vi "Global1.vi"() -> ()   [LabVIEW 2026]
doc: "A global variable which contains communication setup information."
uses:
  Available DLLs.ctl
  Available DLL interfaces.ctl
  Available interfaces.ctl
  Termination character.ctl
  Syntax.ctl
panel:
  in  "DLL path":path
  in  "Error Check":bool[](array[boolean])
  in  "PI Semaphore":string[](array[string])
  out "Log file ref. no":refnum<file>
  in  "Logging mode":bool
  in  "Syntax":T1[](array[typedef])
  in  "Termination character":T2[](array[typedef])
  out "VISA Resource name":refnum<visa-resource-name>[](array[refnum])
  in  "TCP/IP Configuration":T3(array[cluster])
  in  "Bit settings and parity":T4(array[cluster]) {"data bits" min=5 max=8 step=1}
  in  "Flow control":T5(array[cluster]) {"parity error byte" format="%.0x"; "XON byte" format="%.0x"; "XOFF byte" format="%.0x"}
  in  "Interface configuration":T7(array[cluster]) {"Interface" items=["RS232", "GPIB", "DLL", "TCP-IP", "USB", "Analog"]; "RS232 Portnumber" items=["COM1", "COM2", "COM3", "COM4", "COM5", "COM6", "COM7", "COM8", "COM9", "COM10", "COM11", "COM12", "COM13", "COM14", "COM15", "COM16", "COM17", "COM18", "COM19", "COM20", "COM21", "COM22", "COM23", "COM24", "COM25", "COM26", "COM27", "COM28", "COM29", "COM30"]}
  in  "DLL Interface\nConfiguration":T10(array[cluster]) {"DLL for Device" items=["C-843", "C-844", "E-710", "C-843.PM", "C-865", "E-761", "Mercury", "E-755", "E-753", "C-866", "E-712", "E-725", "E-861", "C-867", "E-517", "E-816", "E-709", "PI_GCS2_DLL", "HydraPollux"]; "DLL Interface" items=["RS232", "GPIB", "Board", "TCP-IP", "USB", "RS232_DC", "USB_DC", "TCPIP_DC"]}
  in  "DLL device ID's":i32[](array[numeric])
  in  "Number of\nsystems":i32 min=0 max=20 step=1
  # "Global 1 is a global variable which contains communication setup information."
  # "RMO, GKo, 07/12/18"
  # "TCP/IP:"
  # "General:"
  # "RS232:"
  # "GPIB:"
  # "DLL:"
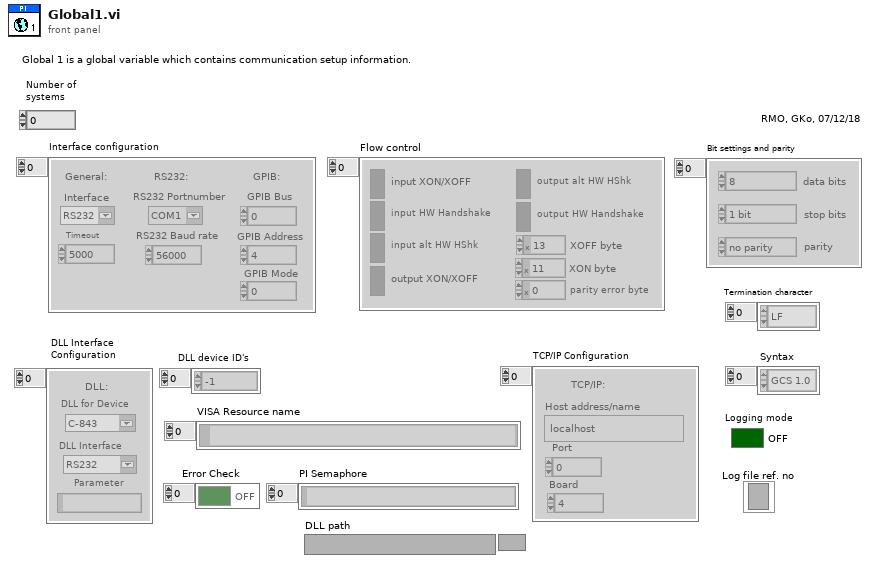
[diagram p1: front panel]
types:
  T1 = typedef "Syntax.ctl" = enum16{"GCS 1.0", "GCS 2.0", "GCS 3.0"}
  T2 = typedef "Termination character.ctl" = enum16{"LF", "CR", "LFCR", "CRLF"}
  T3 = cluster{"Host address/name":string, "Port":i32, "Board":i32}[]
  T4 = cluster{"data bits":u16, "stop bits":enum16{"1 bit", "1.5 bits", "2 bits"}, "parity":enum16{"no parity", "odd parity", "even parity", "mark parity", "space parity"}}[]
  T5 = cluster{"input XON/XOFF":bool, "input HW Handshake":bool, "input alt HW HShk":bool, "output XON/XOFF":bool, "output HW Handshake":bool, "output alt HW HShk":bool, "XOFF byte ":u8, "XON byte":u8, "parity error byte":u16}[]
  T6 = typedef "Available interfaces.ctl" = u16
  T7 = cluster{"RS232 Portnumber":i32, "Timeout":i32, "RS232 Baud rate":u32, "Interface":T6, "GPIB Bus":i32, "GPIB Address":i32, "GPIB Mode":i32}[]
  T8 = typedef "Available DLLs.ctl" = u16
  T9 = typedef "Available DLL interfaces.ctl" = u16
  T10 = cluster{"DLL for Device":T8, "DLL Interface":T9, "Parameter":string}[]
diagram:
